vi "sort.vi"() -> ()   [LabVIEW 2023]
panel:
  out "sorted array":dbl[][](array[numeric]) format="%#_4g"
  out "array":dbl[][](array[numeric]) format="%#_4g"
  in  "columns":dbl
  in  "rows":dbl
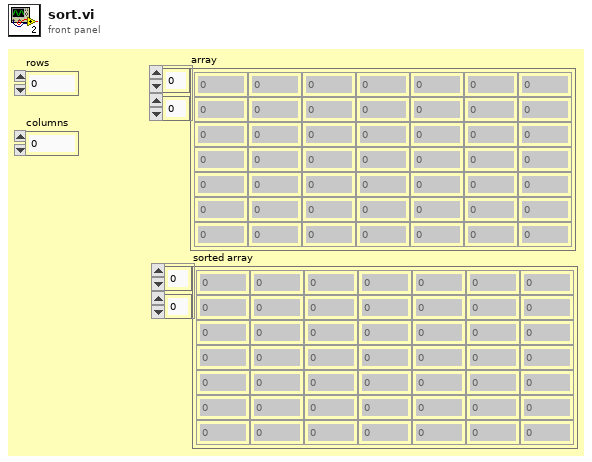
[diagram p1: front panel]
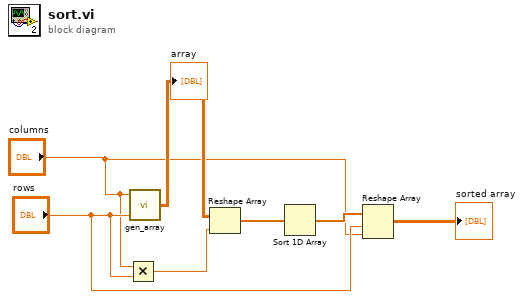
[diagram p0: block diagram]
diagram:
  n1 = Multiply(x="columns", y="rows") -> (x*y=w5:dbl)
  n2 = call "gen_array.vi"("rows"="rows", "columns"="columns") -> ("Array"=w4:dbl[][])
  "array" <- w4
  n3 = Reshape Array(w4, w5) -> (w7:dbl[])
  n4 = Sort 1D Array(array=w7) -> (sorted array=w6:dbl[])
  n5 = Reshape Array(w6, "rows", "columns") -> (→"sorted array":dbl[][])
